vi "ModifyGraph rgb.vi"(8 "error in (no error)":errorcluster, 10 "Colorscale":u32[](array[colorbox])=[16711680, 16744448, 16776960, 65280, 255, 8388863, 16711935], 11 "ITX Commands in":refnum<class "ITX Commands.lvclass">) -> (0 "error out":errorcluster, 3 "ITX Commands out":refnum<class "ITX Commands.lvclass">)   [LabVIEW 2019, in "ITX Commands.lvclass"]
uses:
  ITX Commands.lvclass
  Graph Utilities/graph_utilities.lvclass
panel:
  out "delimited string":string
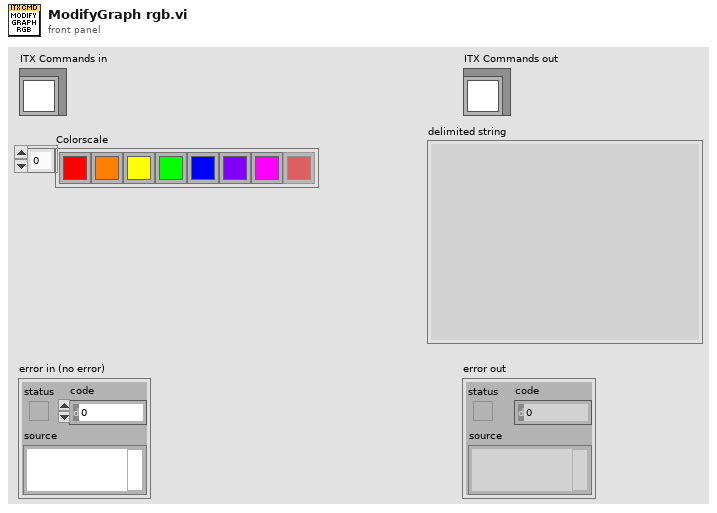
[diagram p1: front panel]
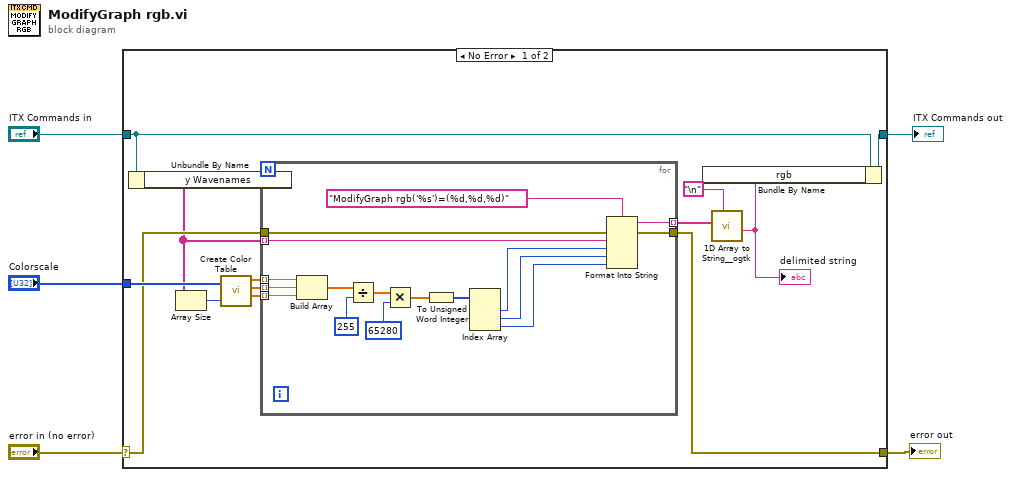
[diagram p0: block diagram]
diagram:
  n1 = case shown="No Error" "error in (no error)" {
    selector: "error in (no error)" -> [w10 w37]
    tunnel: [w9 w37] -> w4
    tunnel: [w15 w36] -> w2
    tunnel: "ITX Commands in" -> [w7 w36]
    tunnel: "Colorscale" -> [w11 _]
    frame No Error {
      n2 = Unbundle By Name(w7) -> ("y Wavenames"=w6:string[])
      n3 = Array Size(array=w6) -> (size(s)=w8:i32)
      n4 = call "Create Color Table.vi"("Colors []"=w11, "Size (256)"=w8) -> ("R []"=w18:dbl[], "G []"=w17:dbl[], "B []"=w16:dbl[])  [unwired: 1 out]
      n5 = for {
        tunnel: w18 -> [w30] mode=indexing
        tunnel: w17 -> [w29] mode=indexing
        tunnel: w16 -> [w28] mode=indexing
        tunnel: [w26] -> w13 mode=indexing
        tunnel: w6 -> [w25] mode=indexing
        tunnel: w10 -> [w20]
        tunnel: [w19] -> w9
        n6 = Build Array(w30, w29, w28) -> (w31:dbl[])
        n7 = Divide(x=w31, y=255) -> (x/y=w32:dbl[])
        n8 = Multiply(x=w32, y=65280) -> (x*y=w33:dbl[])
        n9 = To Unsigned Word Integer(number=w33) -> (unsigned 16bit integer=w24:u16[])
        n10 = Index Array(array=w24) -> (element #1=w23:u16, element #2=w22:u16, element #3=w21:u16)  [unwired: 3 in]
        n11 = Format Into String(format string="ModifyGraph rgb('%s')=(%d,%d,%d)", error in=w20, w25, w23, w22, w21) -> (resulting string=w26:string, error out=w19:errorcluster)  [unwired: 1 in]
      }
      n12 = call "1D Array to String__ogtk.vi"("delimiter (Tab)"="\n", "Array of Strings"=w13) -> ("delimited string"=w12:string)  [unwired: 9 in]
      "delimited string" <- w12
      n13 = Bundle By Name(cluster=w7, "rgb"=w12) -> (w15:refnum<class "ITX Commands.lvclass">)
    }
    frame Error {
    }
  }
  "error out" <- w4
  "ITX Commands out" <- w2
